vi "周期设置_总磷总氮.vi"() -> ()   [LabVIEW 2016, in "斯坦道总氮.lvlib"]
uses:
  <vilib>/Utility/miscctls.llb/LVPointTypeDef.ctl
  <vilib>/ptbypt/NI_PtbyPt.lvlib
panel:
  in  "运行周期":T1={"运行模式"=enum."维护模式", "质控频次"=enum."关闭", "空白核查时间"=2, "跨度核查时间"=6, "测量间隔"=240} {"跨度核查时间" items=["00H", "01H", "02H", "03H", "04H", "05H", "06H", "07H", "08H", "09H", "10H", "11H", "12H", "13H", "14H", "15H", "16H", "17H", "18H", "19H", "20H", "21H", "22H", "23H", "关闭"]; "空白核查时间" items=["00H", "01H", "02H", "03H", "04H", "05H", "06H", "07H", "08H", "09H", "10H", "11H", "12H", "13H", "14H", "15H", "16H", "17H", "18H", "19H", "20H", "21H", "22H", "23H", "关闭"]}
  # "运行模式："
  # "质控频次："
  # "零点核查时间："
  # "跨度核查时间："
  # "测量间隔："
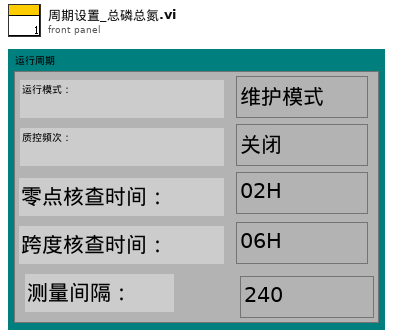
[diagram p1: front panel]
types:
  T1 = cluster{"运行模式":enum16{"维护模式", "常规模式", "应急模式", "质控模式"}, "质控频次":enum16{"关闭", "每天", "星期一", "星期二", "星期三", "星期四", "星期五", "星期六", "星期日"}, "空白核查时间":u16, "跨度核查时间":u16, "测量间隔":u16}
  T2 = typedef "LVPointTypeDef.ctl" = cluster{"Horizontal":i16, "Vertical":i16}
  T3 = typedef "控制命令与参数.ctl" = cluster{"控制命令":enum16{"启动测量", "标样核查", "零点核查", "跨度核查", "空白测试", "平行样测试", "加标回收", "空白校准", "标样校准", "初始化（清洗）", "停止测试", "仪器重启", "校时", "模式设置", "测量间隔设置"}, "测量参数":string}
  T4 = enum16{"启动测量", "标样核查", "零点核查", "跨度核查", "空白测试", "平行样测试", "加标回收", "空白校准", "标样校准", "初始化（清洗）", "停止测试", "仪器重启", "校时", "模式设置", "测量间隔设置"}
  T5 = cluster{"系统时间":timestamp, "工作状态":u16, "测量模式":enum16{"待机", "连续模式", "周期模式", "定点模式", "受控模式", "手动模式"}, "告警代码":u16, "故障代码":u16, "日志代码":u16, "软件版本":u16, "F0":sgl, "F1":sgl, "F2":sgl, "F3":sgl, "T":sgl, "H":sgl, "id":u16, "flowid":u16, "量程":u16, "总磷控温温度1":sgl, "营养盐控温温度2":sgl, "ADC":sgl, "结果值":sgl, "运行时间":u16, "步骤详情":string, "步骤流程":string}
  T6 = enum16{"关闭", "每天", "星期一", "星期二", "星期三", "星期四", "星期五", "星期六", "星期日"}
  T7 = typedef "LVDateTimeRec.ctl" = cluster{"秒数的小数部分":dbl, "秒":i32, "分":i32, "时":i32, "日":i32, "月":i32, "年":i32, "天数（周）":i32, "天数（年）":i32, "DST":i32}
  T8 = cluster{"运行模式":enum16{"维护模式", "常规模式", "应急模式", "质控模式", "性能测试"}, "质控频次":enum16{"关闭", "每天", "星期一", "星期二", "星期三", "星期四", "星期五", "星期六", "星期日"}, "空白核查时间":u16, "跨度核查时间":u16, "测量间隔":u16}
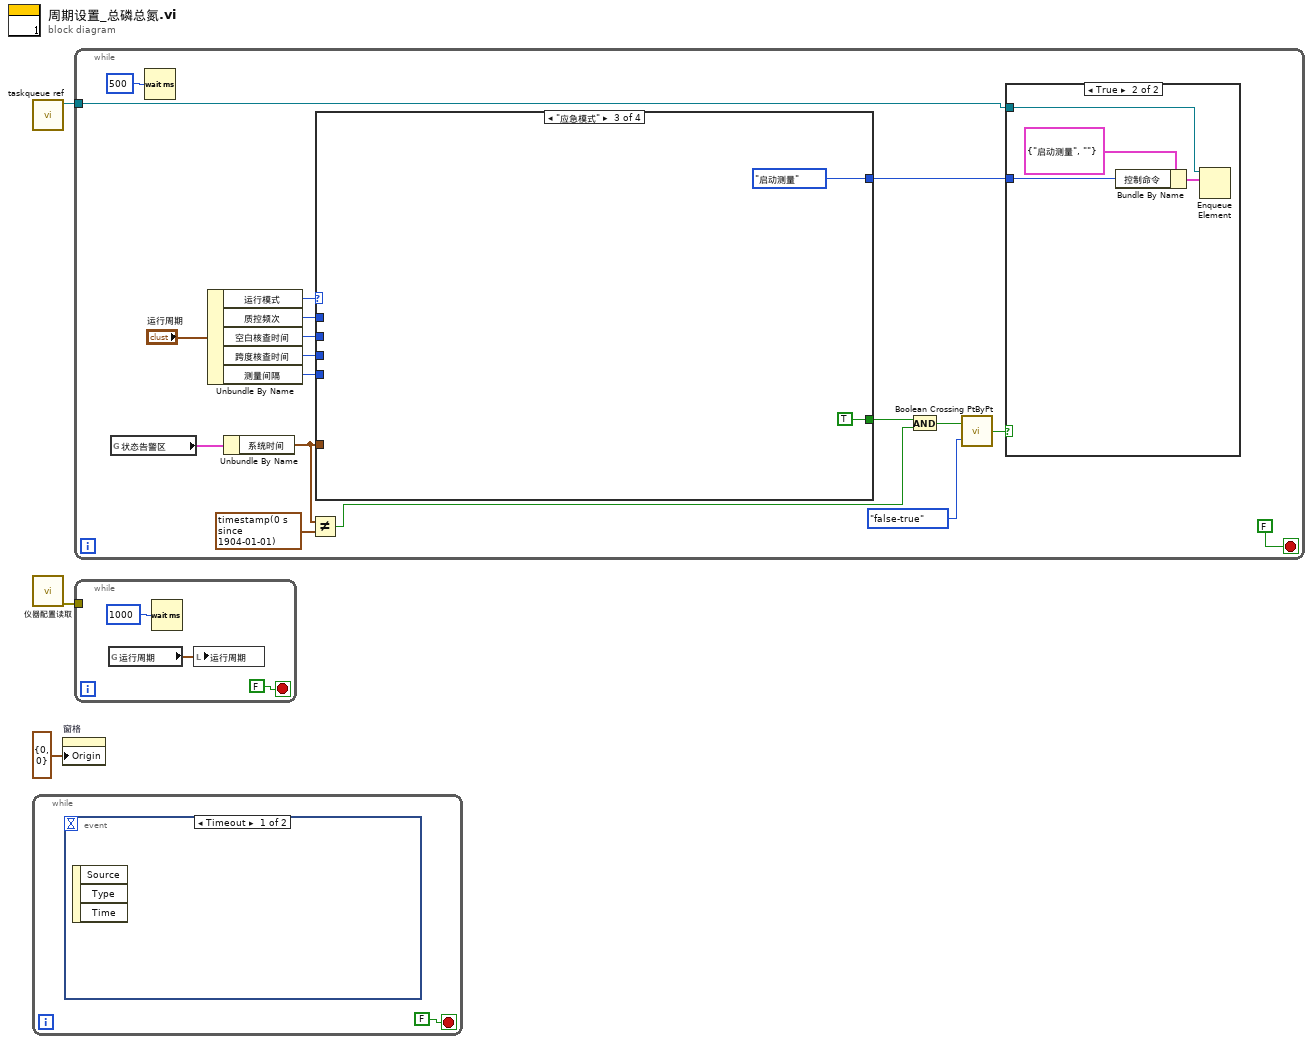
[diagram p0: block diagram]
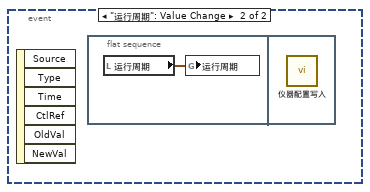
[diagram p2: hidden frame]
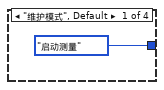
[diagram p4: hidden frame]
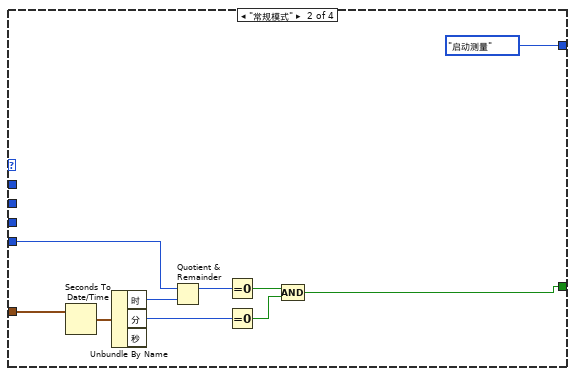
[diagram p5: hidden frame]
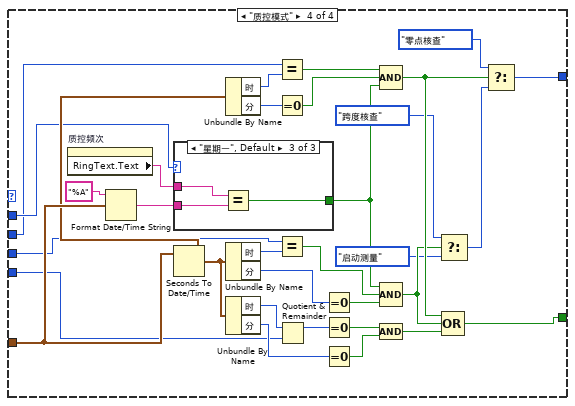
[diagram p6: hidden frame]
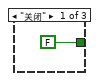
[diagram p7: hidden frame]
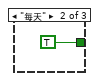
[diagram p8: hidden frame]
diagram:
  n1 = call "taskqueue ref.vi"() -> ("队列输出"=w1:refnum<queue>)  [unwired: 10 in, 1 out]
  n2 = call "仪器配置读取.vi"() -> ("error out"=w2:errorcluster)  [unwired: 11 in]
  n3 = while {
    stop <- FALSE stop-if-true
    n4 = event shown="[0] Timeout" {
      selector: _ -> [_ _]
      dyn-events: _ -> [_ _]
      timeout: _ -> [_ _]
      event Timeout {
        n5 = event-data() -> ()  [unwired: 1 in, 3 out]
      }
      event "运行周期": Value Change {
        n6 = event-data() -> ()  [unwired: 1 in, 6 out]
        n7 = flat-sequence {
          frame #0 {
            n8 = local read "运行周期"() -> (w5:T1)
            n9 = global write "总磷总氮断电保存全局变量.vi" "运行周期"(w5) -> ()
          }
          frame #1 {
            n10 = call "仪器配置写入.vi"() -> ()  [unwired: 11 in, 1 out]
          }
        }
      }
    }
  }
  n11 = property on="窗格" class="Pane"("Origin"=T2 {"Horizontal"=0, "Vertical"=0} ("原点")) -> ()  [unwired: 2 in, 2 out]
  n12 = while {
    tunnel: w1 -> [w8]
    stop <- FALSE stop-if-true
    n13 = global read "VAR总磷总氮全局变量.vi" "状态告警区"() -> (w15:T5)
    n14 = Wait (ms)(milliseconds to wait=u32 500 ("等待时间（毫秒）")) -> ()  [unwired: 1 out]
    n15 = Unbundle By Name("运行周期") -> ("运行模式"=w21:enum16{"维护模式", "常规模式", "应急模式", "质控模式"}, "质控频次"=w20:T6, "空白核查时间"=w19:u16, "跨度核查时间"=w18:u16, "测量间隔"=w17:u16)
    n16 = Unbundle By Name(w15) -> ("系统时间"=w14:timestamp)
    n17 = Not Equal?(x=w14, y=timestamp(0 s since 1904-01-01)) -> (x != y?=w12:bool)
    n18 = case shown="\"应急模式\"" w21 {
      tunnel: w14 -> [_ w38 _ w72]
      tunnel: w17 -> [_ w31 _ w43]
      tunnel: [_ w34 TRUE w58] -> w16
      tunnel: [T4."启动测量" ("控制命令") T4."启动测量" ("控制命令") T4."启动测量" ("控制命令") w54] -> w7
      tunnel: w20 -> [_ _ _ w51]
      tunnel: w19 -> [_ _ _ w50]
      tunnel: w18 -> [_ _ _ w49]
      frame "维护模式", Default {
      }
      frame "常规模式" {
        n19 = Seconds To Date/Time(time stamp (now)=w38) -> (date time rec=w37:T7)  [unwired: 1 in]
        n20 = Unbundle By Name(w37) -> ("时"=w30:i32, "分"=w36:i32)  [unwired: 1 out]
        n21 = Quotient & Remainder(x=w31, y=w30) -> (x-y*floor(x/y)=w32:i32)  [unwired: 1 out]
        n22 = Equal To 0?(x=w32) -> (x = 0?=w29:bool)
        n23 = Equal To 0?(x=w36) -> (x = 0?=w35:bool)
        n24 = Compound Arithmetic op=AND ("复合运算")(w29, w35) -> (w34:bool)
      }
      frame "应急模式" {
      }
      frame "质控模式" {
        n25 = property on="质控频次" class="Enum (strict)"() -> ("RingText.Text"=w45:string)  [unwired: 2 in, 2 out]
        n26 = Format Date/Time String(time format string (%c)="%A" ("时间格式字符串(%c)"), seconds (now)=w72) -> (date/time string=w70:string)  [unwired: 1 in]
        n27 = case shown="\"星期一\", Default" w51 {
          tunnel: w70 -> [_ _ w77]
          tunnel: [FALSE TRUE w76] -> w52
          tunnel: w45 -> [_ _ w75]
          frame "关闭" {
          }
          frame "每天" {
          }
          frame "星期一", Default {
            n28 = Equal?(x=w75, y=w77) -> (x = y?=w76:bool)
          }
        }
        n29 = Seconds To Date/Time(time stamp (now)=w72) -> (date time rec=w61:T7)  [unwired: 1 in]
        n30 = Unbundle By Name(w61) -> ("时"=w67:i32, "分"=w66:i32)
        n31 = Unbundle By Name(w61) -> ("时"=w62:i32, "分"=w63:i32)
        n32 = Unbundle By Name(w61) -> ("时"=w44:i32, "分"=w69:i32)
        n33 = Equal?(x=w50, y=w67) -> (x = y?=w65:bool)
        n34 = Equal To 0?(x=w66) -> (x = 0?=w64:bool)
        n35 = Equal?(x=w49, y=w62) -> (x = y?=w60:bool)
        n36 = Quotient & Remainder(x=w44, y=w43) -> (x-y*floor(x/y)=w42:i32)  [unwired: 1 out]
        n37 = Equal To 0?(x=w63) -> (x = 0?=w59:bool)
        n38 = Equal To 0?(x=w42) -> (x = 0?=w41:bool)
        n39 = Equal To 0?(x=w69) -> (x = 0?=w68:bool)
        n40 = Compound Arithmetic op=AND ("复合运算")(w65, w64, w52) -> (w57:bool)
        n41 = Compound Arithmetic op=AND ("复合运算")(w52, w60, w59) -> (w56:bool)
        n42 = Compound Arithmetic op=AND ("复合运算")(w41, w68) -> (w53:bool)
        n43 = Select(t=T4."跨度核查" ("控制命令"), s=w56, f=T4."启动测量" ("控制命令")) -> (s? t:f=w55:T4)
        n44 = Compound Arithmetic op=OR ("复合运算")(w57, w56, w53) -> (w58:bool)
        n45 = Select(t=T4."零点核查" ("控制命令"), s=w57, f=w55) -> (s? t:f=w54:T4)
      }
    }
    n46 = And(x=w16, y=w12) -> (x .and. y?=w11:bool)
    n47 = call <vilib>:"Boolean Crossing PtByPt.vi"("direction"=enum16{"either", "false-true", "true-false"}."false-true", "input"=w11) -> ("crossing"=w6:bool)  [unwired: 1 in]
    n48 = case shown="True" w6 {
      tunnel: w8 -> [_ w27]
      tunnel: w7 -> [_ w24]
      frame False {
      }
      frame True {
        n49 = Bundle By Name(cluster=T3 {"控制命令"=enum."启动测量", "测量参数"=""} ("element"), "控制命令"=w24) -> (w25:T3)
        n50 = Enqueue Element(queue=w27, element=w25) -> ()  [unwired: 2 in, 3 out]
      }
    }
  }
  n51 = while {
    tunnel: w2 -> [_]
    stop <- FALSE stop-if-true
    n52 = global read "总磷总氮断电保存全局变量.vi" "运行周期"() -> (w78:T8)
    n53 = Wait (ms)(milliseconds to wait=u32 1000 ("等待时间（毫秒）")) -> ()  [unwired: 1 out]
    n54 = local write "运行周期"(w78) -> ()
  }
